vi "Write Text.vi"(8 "error in (no error)":errorcluster, 9 "Text":string, 10 "VISA resource name in":refnum<visa-resource-name>, 11 "LCD-I2C in":refnum<class "LCD-I2C.lvclass">) -> (0 "error out":errorcluster, 2 "VISA resource name":refnum<visa-resource-name>, 3 "LCD-I2C out":refnum<class "LCD-I2C.lvclass">)   [LabVIEW 2023, in "CTI-Visa-DeviceLib.lvlib" / "LCD-I2C.lvclass"]
uses:
  LCD-I2C.lvclass
  LCD-I2C.lvclass/LCD-I2C.ctl
  Mode.ctl
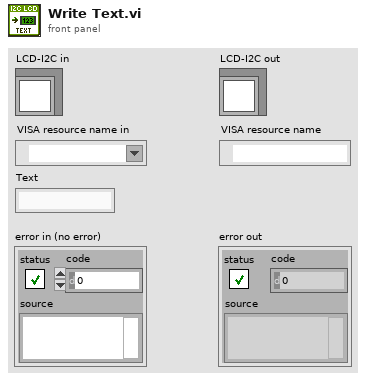
[diagram p1: front panel]
types:
  T1 = typedef "CTI-Visa-DeviceLib.lvlib/LCD-I2C.lvclass/Mode.ctl" = enum8{"Command", "Character"}
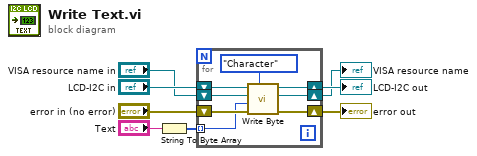
[diagram p0: block diagram]
diagram:
  n1 = String To Byte Array(string="Text") -> (unsigned byte array=w1:u8[])
  n2 = for {
    shift-right: [w15] -> w6
    shift-left: "error in (no error)" -> [w16]
    shift-right: [w13] -> w4
    shift-left: "LCD-I2C in" -> [w14]
    shift-right: [w11] -> w2
    shift-left: "VISA resource name in" -> [w12]
    tunnel: w1 -> [w10] mode=indexing
    n3 = call "Write Byte.vi"("Mode (Command)"=Mode."Character", "error in (no error)"=w16, "Value"=w10, "VISA resource name in"=w12, "LCD-I2C in"=w14) -> ("error out"=w15:errorcluster, "VISA resource name"=w11:refnum<visa-resource-name>, "LCD-I2C out"=w13:refnum<class "LCD-I2C.lvclass">)  [unwired: 4 in]
  }
  "error out" <- w6
  "LCD-I2C out" <- w4
  "VISA resource name" <- w2
